vi "Timer_New.vi"(8 "error in (no error)":errorcluster caption="错误输入（无错误）", 11 "Timer 输入":refnum<class "Timer.lvclass">) -> (0 "error out":errorcluster caption="错误输出", 2 "值引用":refnum<data-value>, 3 "Timer 输出":refnum<class "Timer.lvclass">)   [LabVIEW 2019, in "Timer.lvclass"]
uses:
  Timer.lvclass
  attribute/Attribute.ctl
  Timer.lvclass/Timer.ctl
panel:
  in  "attribute":T1
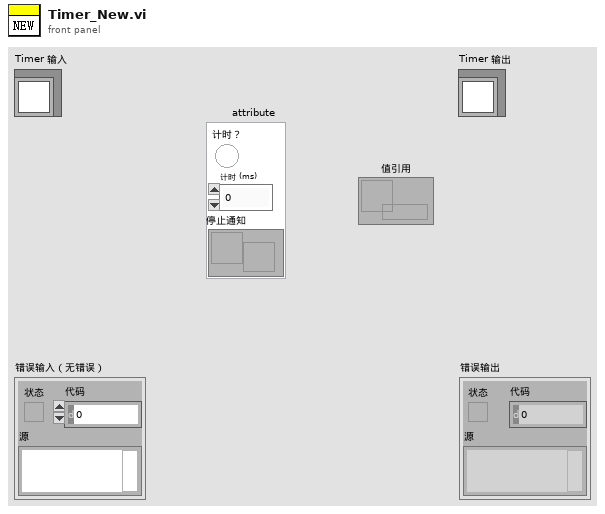
[diagram p1: front panel]
types:
  T1 = typedef "Timer.lvclass/Attribute.ctl" = cluster{"计时？":bool, "计时 (ms)":u32, "停止通知":refnum<notifier>}
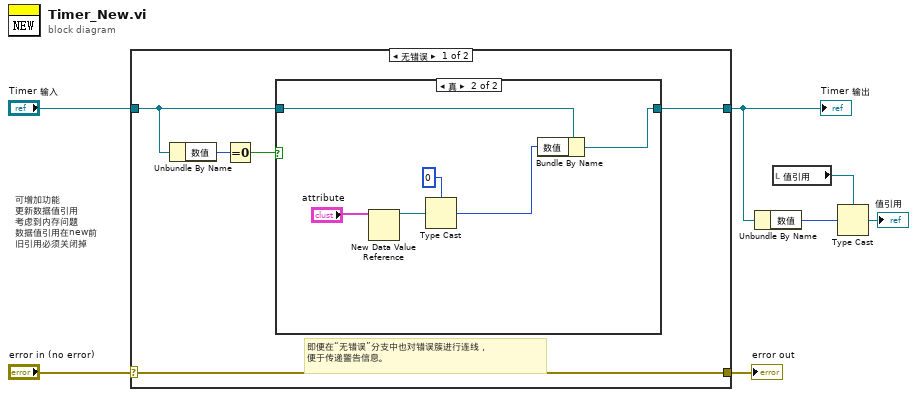
[diagram p0: block diagram]
diagram:
  # "可增加功能\n更新数据值引用\n考虑到内存问题\n数据值引用在new前\n旧引用必须关闭掉"
  n1 = case shown="无错误" "error in (no error)" {
    selector: "error in (no error)" -> [w12 w21]
    tunnel: [w12 w21] -> w6
    tunnel: [w10 w20] -> w4
    tunnel: "Timer 输入" -> [w9 w20]
    frame No Error {
      # "即便在“无错误”分支中也对错误簇进行连线，\n便于传递警告信息。"
      n2 = Unbundle By Name(w9) -> ("数值"=w11:u32)
      n3 = Equal To 0?(x=w11) -> (x = 0?=w8:bool)
      n4 = case shown="真" w8 {
        tunnel: [w13 w14] -> w10
        tunnel: w9 -> [w13 w16]
        frame False {
          # "存在数据值引用，忽略新建操作"
        }
        frame True {
          n5 = New Data Value Reference(data value="attribute") -> (data value reference=w18:refnum<data-value>)  [unwired: 1 in, 1 out]
          n6 = Type Cast(type=u32 0, x=w18) -> (*(type *) &x=w15:u32)
          n7 = Bundle By Name(cluster=w16, "数值"=w15) -> (w14:refnum<class "Timer.lvclass">)
        }
      }
    }
    frame Error {
    }
  }
  "error out" <- w6
  "Timer 输出" <- w4
  n8 = Unbundle By Name(w4) -> ("数值"=w3:u32)
  n9 = local read "值引用"() -> (w1:refnum<data-value>)
  n10 = Type Cast(type=w1, x=w3) -> (*(type *) &x=→"值引用":refnum<data-value>)
